vi "Set Debounce Period.vi"(8 "error in (no error)":errorcluster, 10 "debounce (100)":u32=100, 11 "Ambient Light Bricklet in":refnum<class "Ambient Light Bricklet.lvclass">) -> (0 "error out":errorcluster, 3 "Ambient Light Bricklet out":refnum<class "Ambient Light Bricklet.lvclass">)   [LabVIEW 2011, in "Tinkerforge.lvlib" / "Ambient Light Bricklet.lvclass"]
doc: "This VI sets the debounce period of the callbacks. This period is used if the threshold configuration leads to initial triggering of the callback."
uses:
  Ambient Light Bricklet.lvclass
  Device/Device.lvclass
  IP Connection/IP Connection.lvclass
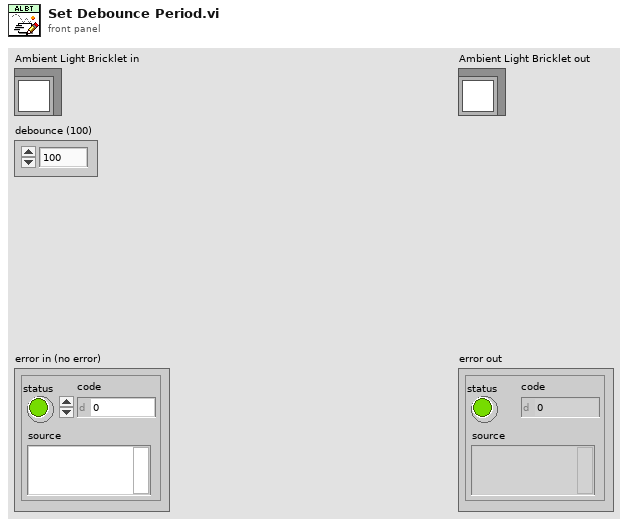
[diagram p1: front panel]
types:
  T1 = enum16{"big-endian, network order", "native, host order", "little-endian"}
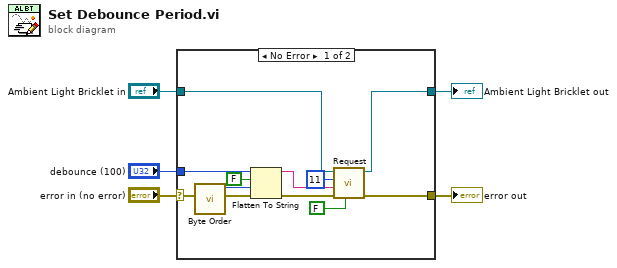
[diagram p0: block diagram]
diagram:
  n1 = case shown="No Error" "error in (no error)" {
    selector: "error in (no error)" -> [w11 w18]
    tunnel: [w12 w18] -> w4
    tunnel: [w15 w17] -> w2
    tunnel: "Ambient Light Bricklet in" -> [w16 w17]
    tunnel: "debounce (100)" -> [w8 _]
    frame No Error {
      n2 = call "Byte Order.vi"() -> ("byte order (2:little-endian)"=w6:T1)  [unwired: 11 in]
      n3 = Flatten To String(anything=w8, prepend array or string size? (T)=FALSE, byte order (0:big-endian, network order)=w6, error in (no error)=w11) -> (data string=w9:string, error out=w10:errorcluster)  [unwired: 1 out]
      n4 = call "Request.vi"("Response"=FALSE, "error in (no error)"=w10, "Data"=w9, "Function ID"=u8 11, "Device in"=w16) -> ("error out"=w12:errorcluster, "Device out"=w15:refnum<class "Ambient Light Bricklet.lvclass">)  [unwired: 2 in, 3 out]
    }
    frame Error {
    }
  }
  "error out" <- w4
  "Ambient Light Bricklet out" <- w2
